vi "test.vi"   [LabVIEW 2021]
uses:
  CBar/CBar.lvclass
  CFoo/CFoo.lvclass
  IBBB/IBBB.lvclass
  IAAA/IAAA.lvclass
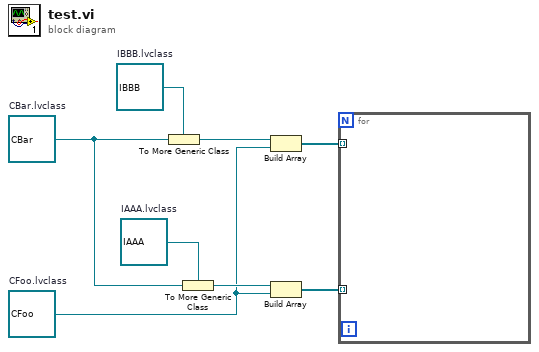
[diagram p0: block diagram]
diagram:
  w8 = refnum<class "IAAA.lvclass"> refnum  # IAAA.lvclass
  w7 = refnum<class "IBBB.lvclass"> refnum  # IBBB.lvclass
  w3 = refnum<class "CFoo.lvclass"> refnum  # CFoo.lvclass
  w6 = refnum<class "CBar.lvclass"> refnum  # CBar.lvclass
  n1 = To More Generic Class(target class=w7, reference=w6) -> (generic class reference=w4:refnum<class "IBBB.lvclass">)
  n2 = To More Generic Class(target class=w8, reference=w6) -> (generic class reference=w5:refnum<class "IAAA.lvclass">)
  n3 = Build Array(w4, w3) -> (w1:refnum<class "IBBB.lvclass">[])
  n4 = Build Array(w5, w3) -> (w2:refnum<class "IAAA.lvclass">[])
  n5 = for {
    tunnel: w2 -> [_] mode=indexing
    tunnel: w1 -> [_] mode=indexing
  }
